vi "RemoveOffset.vi"(10 "offset value":dbl format="%#_13g", 11 "waveform":waveform(dbl)) -> (3 "output waveform":waveform(dbl))   [LabVIEW 2025]
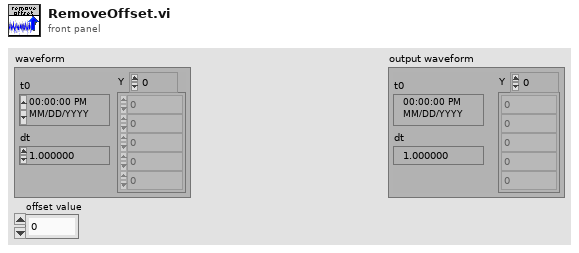
[diagram p1: front panel]
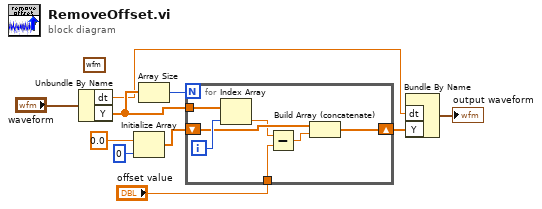
[diagram p0: block diagram]
diagram:
  (unwired) waveform(dbl) {"t0"=timestamp(0 s since 1904-01-01), "dt"=1.0, "Y"=[]} ("Waveform")
  n1 = Unbundle By Name("waveform") -> ("dt"=w3:dbl, "Y"=w9:dbl[])
  n2 = Initialize Array(0.0 ("element"), 0 ("dimension size")) -> (w5:dbl[])
  n3 = Array Size(array=w9) -> (size(s)=w10:i32)
  n4 = for {
    N: w10 -> [_]
    tunnel: w9 -> [w16]
    shift-right: [w14] -> w2
    shift-left: w5 -> [w15]
    tunnel: "offset value" -> [w12]
    i -> [w17]
    n5 = Index Array(array=w16, index=w17) -> (element=w13:dbl)
    n6 = Subtract(x=w13, y=w12) -> (x-y=w11:dbl)
    n7 = Build Array (concatenate)(w15, w11) -> (w14:dbl[])
  }
  n8 = Bundle By Name("dt"=w3, "Y"=w2) -> (→"output waveform":waveform(dbl))  [unwired: 1 in]
